vi "Add Multiple Headers.vi"(8 "error in":errorcluster, 10 "headers":cluster{"header":string, "value":string}[](array[cluster]), 11 "net-http-client in":refnum<class "net-http-client.lvclass">) -> (0 "error out":errorcluster, 3 "net-http-client out":refnum<class "net-http-client.lvclass">)   [LabVIEW 2020, in "net-http-client.lvclass"]
uses:
  net-http-client.lvclass
  net-http-client.lvclass/net-http-client.ctl
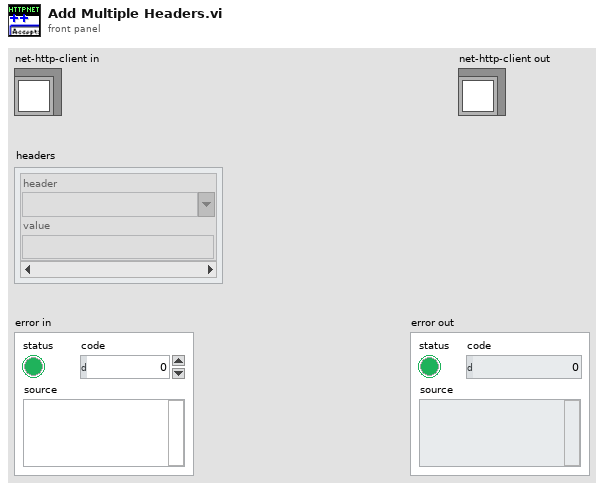
[diagram p1: front panel]
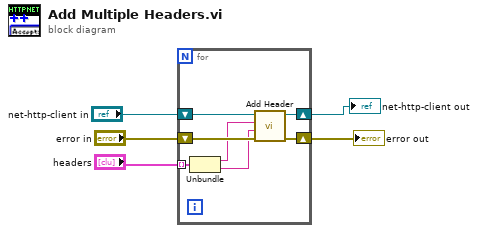
[diagram p0: block diagram]
diagram:
  n1 = for {
    shift-right: [w11] -> w4
    shift-left: "error in" -> [w12]
    shift-right: [w9] -> w2
    shift-left: "net-http-client in" -> [w10]
    tunnel: "headers" -> [w8] mode=indexing
    n2 = Unbundle(w8) -> ("header"=w7:string, "value"=w6:string)
    n3 = call-dynamic "Add Header.vi"("error in"=w12, "value"=w6, "header"=w7, "net-http-client in"=w10) -> ("error out"=w11:errorcluster, "net-http-client out"=w9:refnum<class "net-http-client.lvclass">)  [unwired: 6 in]
  }
  "error out" <- w4
  "net-http-client out" <- w2
